vi "TCL Log Event to Disk.vi"(0 "Event":string[](array[string])) -> ()   [LabVIEW 2009]
uses:
  TCL Global.vi
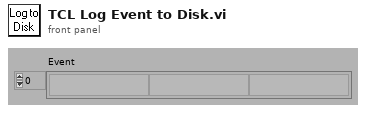
[diagram p1: front panel]
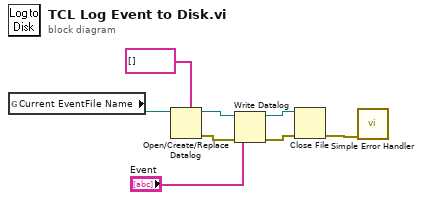
[diagram p0: block diagram]
diagram:
  n1 = global read "TCL Global.vi" "Current EventFile Name"() -> (w5:path)
  n2 = Open/Create/Replace Datalog(5:string[] [], 11:w5) -> (0:w4:errorcluster, 3:w8:refnum<k1>)  [unwired: 4 in, 1 out]
  n3 = Write Datalog(4:w4, 6:"Event", 7:w8) -> (0:w3:errorcluster, 3:w7:refnum<k1>)
  n4 = Close File(refnum=w7, error in=w3) -> (error out=w2:errorcluster)  [unwired: 1 out]
  n5 = call <vilib>:"Simple Error Handler.vi"("error in (no error)"=w2) -> ()  [unwired: 4 in, 5 out]
